vi "Exponential Fit.vi"(0 "Y":dbl[](array[numeric]), 5 "X":dbl[](array[numeric]), 7 "Weight":dbl[](array[numeric]), 9 "tolerance":dbl=0.0001 format="%#_3g", 11 "method":T2 items=["Least Square", "Least Absolute Residual", "Bisquare"], 12 "parameter bounds":T1={"amp min"=-inf, "amp max"=inf, "damping min"=-inf, "damping max"=inf, "offset min"=0.0, "offset max"=0.0}) -> (4 "Best Exponential Fit":dbl[](array[numeric]), 6 "amplitude":dbl, 8 "damping":dbl, 10 "offset":dbl, 14 "residue":dbl, 15 "error":i32)   [LabVIEW 2017, in "NI_AALPro.lvlib"]
doc: "Returns the exponential fit of a data set (<B>X</B>, <B>Y</B>) using the Least Square, Least Absolute Residual, or Bisquare method."
uses:
  NI_AALPro.lvlib
  Curve Fitting Criteria.ctl
  lvanlys.dll
panel:
  # "Constrained Exponential Fit"
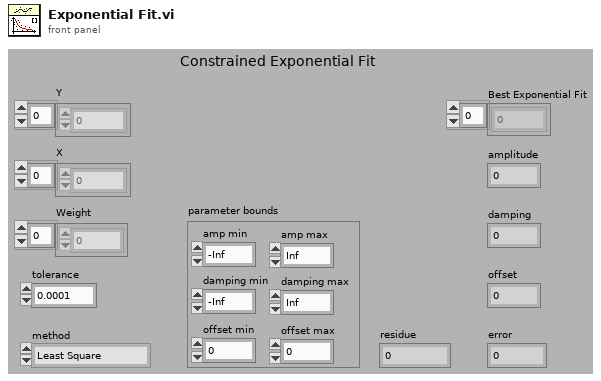
[diagram p1: front panel]
types:
  T1 = cluster{"amp min":dbl, "amp max":dbl, "damping min":dbl, "damping max":dbl, "offset min":dbl, "offset max":dbl}
  T2 = typedef "NI_AALPro.lvlib/Curve Fitting Criteria.ctl" = u16
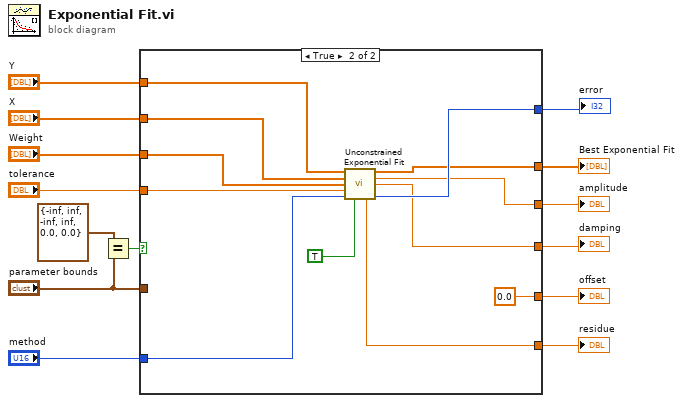
[diagram p0: block diagram]
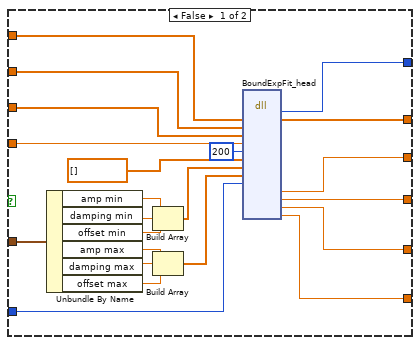
[diagram p2: hidden frame]
diagram:
  n1 = Equal?(x=T1 {"amp min"=-inf, "amp max"=inf, "damping min"=-inf, "damping max"=inf, "offset min"=0.0, "offset max"=0.0} ("parameter bounds 2"), y="parameter bounds") -> (x = y?=w1:bool)
  n2 = case shown="True" w1 {
    tunnel: "Y" -> [w36 w47]
    tunnel: "X" -> [w35 w46]
    tunnel: "Weight" -> [w34 w45]
    tunnel: "tolerance" -> [w33 w44]
    tunnel: "method" -> [w31 w48]
    tunnel: [w29 w42] -> w9
    tunnel: [w28 w41] -> w8
    tunnel: [w27 0.0 ("offset")] -> w7
    tunnel: [w26 w38] -> w6
    tunnel: [w25 w40] -> w5
    tunnel: [w24 w43] -> w4
    tunnel: "parameter bounds" -> [w15 _]
    frame False {
      n3 = Unbundle By Name(w15) -> ("amp min"=w23:dbl, "damping min"=w22:dbl, "offset min"=w21:dbl, "amp max"=w19:dbl, "damping max"=w18:dbl, "offset max"=w17:dbl)
      n4 = Build Array(w23, w22, w21) -> (w20:dbl[])
      n5 = Build Array(w19, w18, w17) -> (w16:dbl[])
      n6 = dll-call lib="C:/Program Files/National Instruments/LabVIEW 2017/resource/lvanlys.*" fn="BoundExpFit_head"("y"=w36, "x"=w35, "weight"=w34, "tolerance"=w33, "maxIter"=200, "intial coef"=dbl[] [], "minBound"=w20, "maxBound"=w16, "algorithm"=w31) -> ("return type"=w24:i32, "y"=w29:dbl[], "amp"=w28:dbl, "damping"=w25:dbl, "offset"=w27:dbl, "mse"=w26:dbl)  [unwired: 9 in, 8 out]
    }
    frame True {
      n7 = call "Unconstrained Exponential Fit.vi"("Y"=w47, "X"=w46, "Weight"=w45, "tolerance"=w44, "method"=w48, "refine?"=TRUE) -> ("Best Exponential Fit"=w42:dbl[], "amplitude"=w41:dbl, "damping"=w40:dbl, "residue"=w38:dbl, "error"=w43:i32)  [unwired: 5 out]
    }
  }
  "error" <- w4
  "Best Exponential Fit" <- w9
  "residue" <- w6
  "amplitude" <- w8
  "offset" <- w7
  "damping" <- w5
